vi "Hitrap_DiagnosticBoxGUI.config controls.vi"(1 "Text":string, 8 "Refnum GO-Control":refnum<vi>, 9 "Refnum Pos Reached Control":refnum<vi>) -> ()   [LabVIEW 2014, in "Hitrap_DiagnosticBoxGUI.lvlib"]
doc: "Configured the reference button. Writes the Diagnostic name on the button or disable it."
uses:
  Hitrap_DiagnosticBoxGUI.lvlib
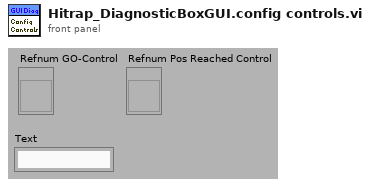
[diagram p1: front panel]
types:
  T1 = enum8{"Enabled", "Disabled", "Disabled and Grayed Out"}
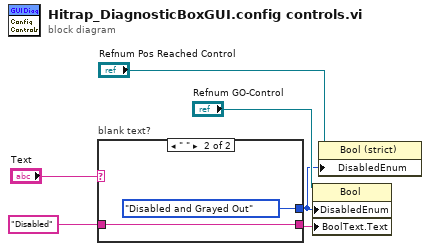
[diagram p0: block diagram]
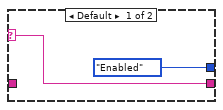
[diagram p2: hidden frame]
diagram:
  n1 = case "blank text?" shown="\" \"" "Text" {
    selector: "Text" -> [w8 _]
    tunnel: [w8 w10] -> w6
    tunnel: "Disabled" -> [_ w10]
    tunnel: [T1."Enabled" ("Disabled") T1."Disabled and Grayed Out" ("Disabled")] -> w2
    frame Default {
    }
    frame " " {
    }
  }
  n2 = property on="Property Node" class="Bool"(reference="Refnum GO-Control", "DisabledEnum"=w2, "BoolText.Text"=w6) -> ()  [unwired: 1 in, 2 out]
  n3 = property on="Property Node" class="Bool (strict)"(reference="Refnum Pos Reached Control", "DisabledEnum"=w2) -> ()  [unwired: 1 in, 2 out]
